vi "exam.vi"() -> ()   [LabVIEW 2021]
uses:
  ae7a6dcb-4cd7-45a0-a870-6559d683a074.vi
  <vilib>/express/express analysis/Spectral/Block/exnSpectralBlock spectral measurements RMS poly.vi
  <vilib>/express/express analysis/Spectral/Block/exnSpectralBlock spectral measurements RMS DDT.vi
  <vilib>/measure/madcrms.llb/Basic Averaged DC-RMS for 1 Chan.vi
  <vilib>/express/express analysis/Spectral/Block/exnSpectralBlock spectral measurements peak poly.vi
  <vilib>/express/express analysis/Spectral/Block/exnSpectralBlock spectral measurements peak WFM.vi
  <vilib>/express/express analysis/Spectral/XNode/ExpressSpectralMeasurementsBlockNode.xnode
  <vilib>/Comparison/Less/Less Functor/Less Functor.lvclass
  <vilib>/measure/NI_MAPro.lvlib
panel:
  out "Array 4":dbl[](array[numeric])
  out "max index(es)":i32
  out "max value 2":dbl
  out "harmonik sum 2":dbl
  out "max noise":dbl
  in  "Boolean":bool
  out "enob 2":dbl
  out "frq 2":dbl
  out "amp":dbl
  out "enob":dbl
  out "Array 3":dbl[][](array[numeric])
  out "Array 2":i32[](array[numeric])
  out "max value":dbl
  out "Array":dbl[](array[numeric])
  out "sınad":dbl
  out "thd (db)":dbl
  out "vrms noise 2":dbl
  out "V fund":dbl
  in  "array size":i32
  out "v rms signal":dbl
  out "vrms max noise":dbl
  out "fft - signal and harmonic":waveform(dbl)(graph)
  out "fft p-p db":cluster{"f0":dbl, "df":dbl, "magnitude":dbl[]}(graph)
  out "SNR":dbl
  out "SFDR":dbl
  out "size  fft":dbl
  out "FUNDAMENTAL":dbl
  out "DF":dbl
  out "fft":dynamicdata(graph)
  out "signal":dynamicdata(graph)
  in  "rate":dbl=1000.0
  in  "number of samples":i32=1000
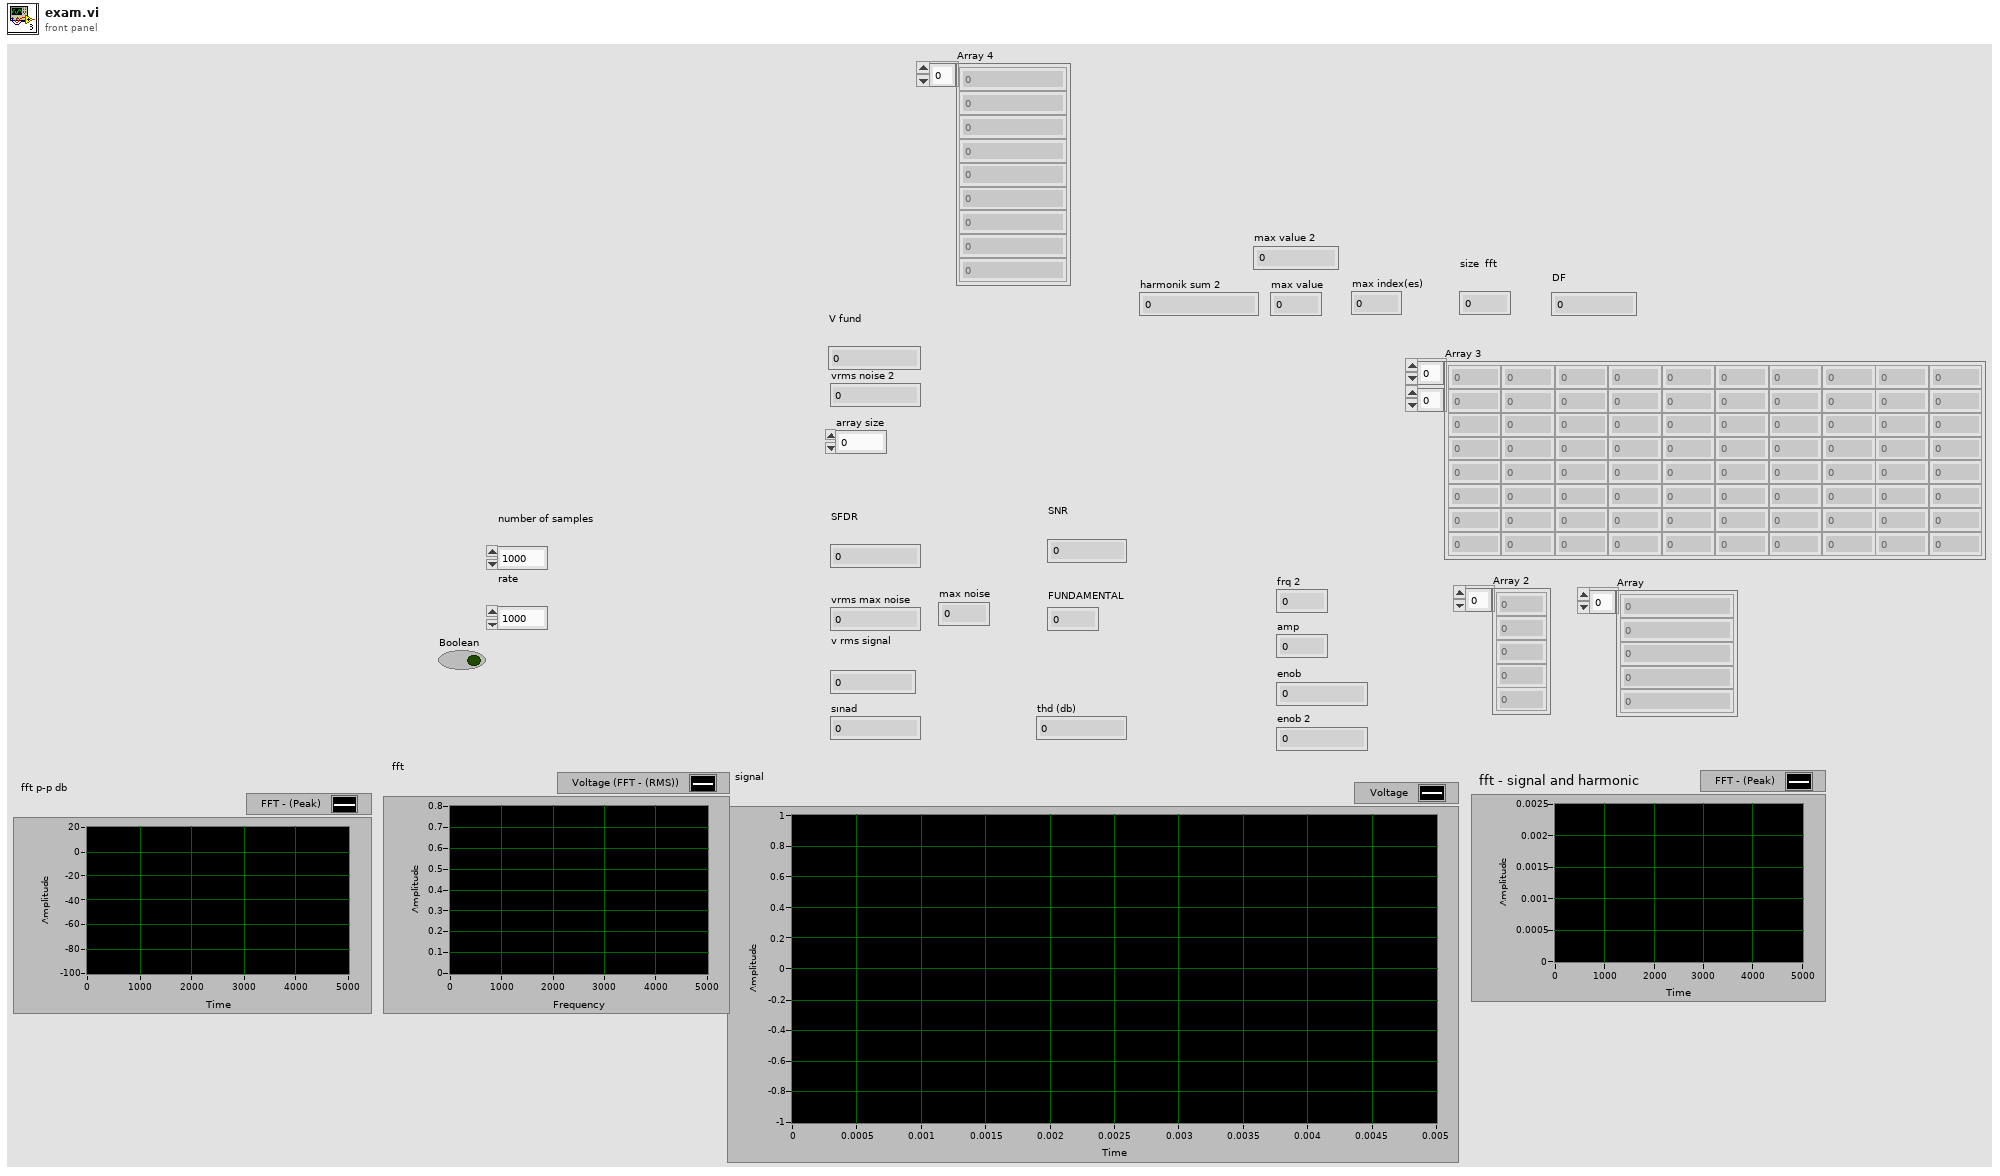
[diagram p1: front panel]
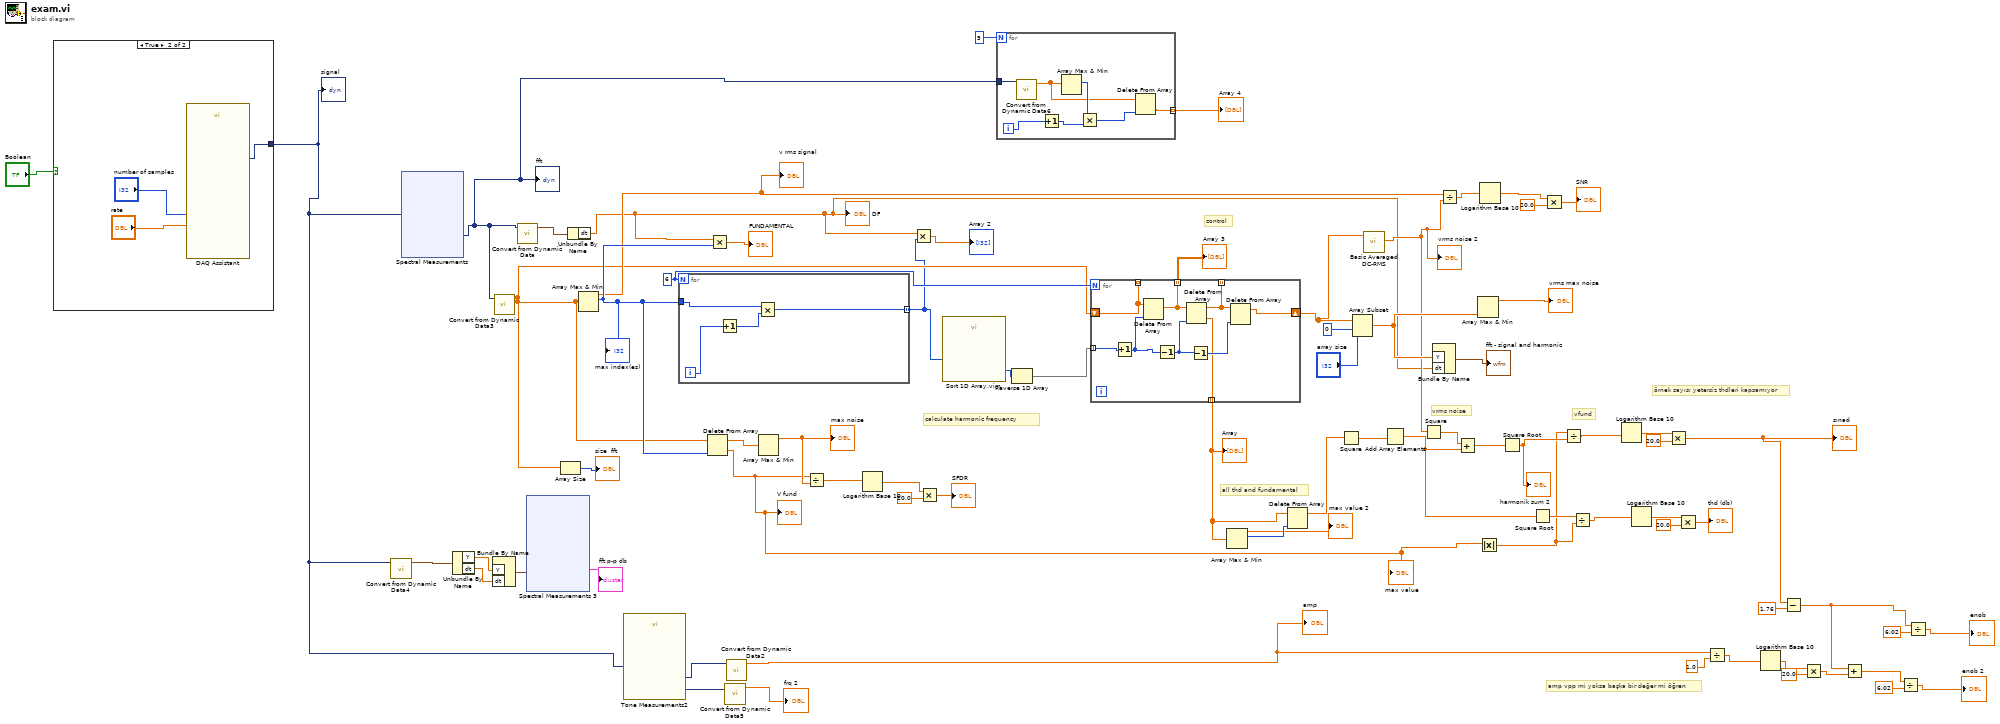
[diagram p0: block diagram]
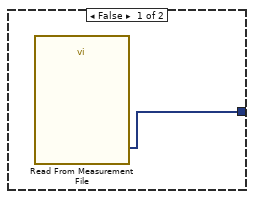
[diagram p2: hidden frame]
diagram:
  w60 = 6
  # "calculate harmonic frequency"
  # "amp vpp mi yoksa başka bir değer mi öğren"
  # "örnek sayısı yetersiz thdleri kapsamıyor"
  # "control"
  # "vfund"
  # "vrms noise"
  # "all thd and fundamental"
  n1 = case shown="True" "Boolean" {
    tunnel: [w77 w80] -> w7
    frame False {
      n2 = call "Read From Measurement File"() -> ("Signals"=w77:dynamicdata)  [unwired: 6 in, 5 out]
    }
    frame True {
      n3 = call "DAQ Assistant"("rate"="rate", "number of samples"="number of samples") -> ("data"=w80:dynamicdata)  [unwired: 15 in, 2 out]
    }
  }
  "signal" <- w7
  n4 = call "Convert from Dynamic Data4"("Dynamic Data Type"=w7) -> ("Waveform"=w9:waveform(dbl))  [unwired: 3 in]
  n5 = xnode "Spectral Measurements"("Signals"=w7) -> ("FFT - (RMS)"=w2:dynamicdata)  [unwired: 1 in, 2 out]
  "fft" <- w2
  n6 = Unbundle By Name(w9) -> ("Y"=w63:dbl[], "dt"=w10:dbl)
  n7 = Bundle By Name("Y"=w63, "dt"=w10) -> (w62:waveform(dbl))  [unwired: 1 in]
  n8 = call "Convert from Dynamic Data3"("Dynamic Data Type"=w2) -> ("Array"=w8:dbl[])  [unwired: 3 in]
  n9 = call "Convert from Dynamic Data"("Dynamic Data Type"=w2) -> ("Waveform"=w76:waveform(dbl))  [unwired: 3 in]
  n10 = xnode "Spectral Measurements 3"("Signals"=w62) -> ("FFT - (Peak)"=→"fft p-p db":cluster{"f0":dbl, "df":dbl, "magnitude":dbl[]})  [unwired: 1 in, 2 out]
  n11 = Array Size(array=w8) -> (size(s)=→"size  fft":i32)
  n12 = Unbundle By Name(w76) -> ("dt"=w5:dbl)
  "DF" <- w5
  n13 = Array Max & Min(array=w8) -> (max value=w56:dbl, max index (indices)=w61:i32)  [unwired: 2 out]
  "v rms signal" <- w56
  "max index(es)" <- w61
  n14 = call "Tone Measurements2"("Signals"=w7) -> ("Frequency"=w33:dynamicdata, "Amplitude"=w34:dynamicdata)  [unwired: 8 in, 1 out]
  n15 = for {
    N: w60 -> [_]
    tunnel: w61 -> [w84]
    tunnel: [w81] -> w6 mode=indexing
    i -> [w82]
    n16 = Increment(x=w82) -> (x+1=w83:i32)
    n17 = Multiply(x=w84, y=w83) -> (x*y=w81:i32)
  }
  n18 = Delete From Array(array=w8, index=w61) -> (deleted portion=w11:dbl, array with subset deleted=w73:dbl[])  [unwired: 1 in]
  "V fund" <- w11
  "max value" <- w11
  n19 = Multiply(x=w5, y=w61) -> (x*y=→"FUNDAMENTAL":dbl)
  n20 = call "Convert from Dynamic Data5"("Dynamic Data Type"=w33) -> ("Scalar"=→"frq 2":dbl)  [unwired: 3 in]
  n21 = call "Convert from Dynamic Data2"("Dynamic Data Type"=w34) -> ("Scalar"=w27:dbl)  [unwired: 3 in]
  "amp" <- w27
  n22 = Array Max & Min(array=w73) -> (max value=w54:dbl)  [unwired: 3 out]
  "max noise" <- w54
  n23 = Divide(x=w11, y=w54) -> (x/y=w72:dbl)
  n24 = Logarithm Base 10(1:w72) -> (0:w71:dbl)
  n25 = Multiply(x=w5, y=w6) -> (x*y=→"Array 2":dbl[])
  n26 = Multiply(x=w71, y=20.0) -> (x*y=→"SFDR":dbl)
  n27 = call "Sort 1D Array.vim"("unsorted array"=w6) -> ("sorted array"=w38:i32[])  [unwired: 10 in]
  n28 = for {
    N: 5 -> [_]
    tunnel: w2 -> [w89]
    tunnel: [w85] -> w1 mode=indexing
    i -> [w88]
    n29 = call "Convert from Dynamic Data6"("Dynamic Data Type"=w89) -> ("Array"=w86:dbl[])  [unwired: 3 in]
    n30 = Increment(x=w88) -> (x+1=w87:i32)
    n31 = Array Max & Min(array=w86) -> (max index (indices)=w91:i32)  [unwired: 3 out]
    n32 = Multiply(x=w91, y=w87) -> (x*y=w90:i32)
    n33 = Delete From Array(array=w86, index=w90) -> (deleted portion=w85:dbl)  [unwired: 1 in, 1 out]
  }
  "Array 4" <- w1
  n34 = Reverse 1D Array(array=w38) -> (reversed array=w37:i32[])
  n35 = for {
    N: w60 -> [_]
    tunnel: w37 -> [w100] mode=indexing
    tunnel: [w96] -> w51 mode=indexing
    tunnel: [w93] -> _ mode=indexing
    tunnel: [w95] -> w36 mode=indexing
    tunnel: [w94] -> _ mode=indexing
    shift-right: [w92] -> w35
    shift-left: w8 -> [w93]
    n36 = Increment(x=w100) -> (x+1=w99:i32)
    n37 = Delete From Array(array=w93, index=w99) -> (array with subset deleted=w95:dbl[])  [unwired: 1 in, 1 out]
    n38 = Decrement(x=w99) -> (x-1=w98:i32)
    n39 = Delete From Array(array=w95, index=w98) -> (deleted portion=w96:dbl, array with subset deleted=w94:dbl[])  [unwired: 1 in]
    n40 = Decrement(x=w98) -> (x-1=w97:i32)
    n41 = Delete From Array(array=w94, index=w97) -> (array with subset deleted=w92:dbl[])  [unwired: 1 in, 1 out]
  }
  "Array" <- w51
  "Array 3" <- w36
  n42 = Array Max & Min(array=w51) -> (max value=→"max value 2":dbl, max index (indices)=w52:i32)  [unwired: 2 out]
  n43 = Delete From Array(array=w51, index=w52) -> (array with subset deleted=w49:dbl[])  [unwired: 1 in, 1 out]
  n44 = Square(x=w49) -> (x^2=w50:dbl[])
  n45 = Array Subset(array=w35, index=0, length="array size") -> (w53:dbl[])
  n46 = call-poly <vilib>:"Basic Averaged DC-RMS.vi"("signal in"=w35) -> ("RMS value"=w12:dbl)  [unwired: 7 in, 3 out]
  "vrms noise 2" <- w12
  n47 = Add Array Elements(numeric array=w50) -> (sum=w40:dbl)
  n48 = Square(x=w12) -> (x^2=w41:dbl)
  n49 = Bundle By Name("Y"=w53, "dt"=w5) -> (→"fft - signal and harmonic":waveform(dbl))  [unwired: 1 in]
  n50 = Divide(x=w56, y=w12) -> (x/y=w67:dbl)
  n51 = Add(x=w41, y=w40) -> (x+y=w39:dbl)
  n52 = Array Max & Min(array=w53) -> (max value=→"vrms max noise":dbl)  [unwired: 3 out]
  n53 = Absolute Value(x=w11) -> (abs(x)=w14:dbl)
  n54 = Logarithm Base 10(1:w67) -> (0:w66:dbl)
  n55 = Square Root(x=w39) -> (sqrt(x)=w15:dbl)
  "harmonik sum 2" <- w15
  n56 = Square Root(x=w40) -> (sqrt(x)=w48:dbl)
  n57 = Multiply(x=w66, y=20.0) -> (x*y=→"SNR":dbl)
  n58 = Divide(x=w14, y=w15) -> (x/y=w16:dbl)
  n59 = Divide(x=w48, y=w14) -> (x/y=w47:dbl)
  n60 = Logarithm Base 10(1:w16) -> (0:w43:dbl)
  n61 = Logarithm Base 10(1:w47) -> (0:w46:dbl)
  n62 = Multiply(x=w43, y=20.0) -> (x*y=w30:dbl)
  "sınad" <- w30
  n63 = Multiply(x=w46, y=20.0) -> (x*y=→"thd (db)":dbl)
  n64 = Divide(x=w27, y=1.0) -> (x/y=w25:dbl)
  n65 = Logarithm Base 10(1:w25) -> (0:w24:dbl)
  n66 = Subtract(x=w30, y=1.76) -> (x-y=w22:dbl)
  n67 = Multiply(x=w24, y=20.0) -> (x*y=w21:dbl)
  n68 = Add(x=w22, y=w21) -> (x+y=w18:dbl)
  n69 = Divide(x=w18, y=6.02) -> (x/y=→"enob 2":dbl)
  n70 = Divide(x=w22, y=6.02) -> (x/y=→"enob":dbl)
